vi "RX IQ Processing.vi"(0 "configuration":T4={"primary channel selector"=0.0, "last OFDM symbol index"=0, "switch format detection states"=TRUE, "format"=enum."NON_HT_OFDM", "bandwidth"=enum."20MHz"}, 1 "packet start":bool, 5 "channels in":T2, 9 "input valid":bool) -> (3 "primary channel selector":fxp<+,2,0>, 4 "last OFDM symbol index":u16, 6 "subcarrier index unsigned":u8, 8 "channel estimate timing":T3, 10 "channel estimate":T1, 12 "last sample":bool, 13 "subcarrier index":fxp<+/-,9,9>, 15 "output valid":bool=TRUE)   [LabVIEW 2020]
uses:
  Configuration Control.ctl
panel:
  out "subcarrier channel 2.Imag":fxp<+/-,25,4>
  out "subcarrier channel.Real":fxp<+/-,25,4>
  out "OFDM symbol start 2":bool
  out "packet_start 2":bool
  out "valid 2":bool
  out "OFDM symbol index 2":u16
  out "sample index 2":u16
  out "Imag 4":fxp<+/-,16,3>
  out "Real 4":fxp<+/-,16,3>
  out "OFDM symbol start":bool
  out "packet_start":bool
  out "valid":bool
  out "OFDM symbol index":u16
  out "sample index":u16
  out "Imag 3":fxp<+/-,16,3>
  out "Real 3":fxp<+/-,16,3>
  out "Imag 2":fxp<+/-,16,3>
  out "Real 2":fxp<+/-,16,3>
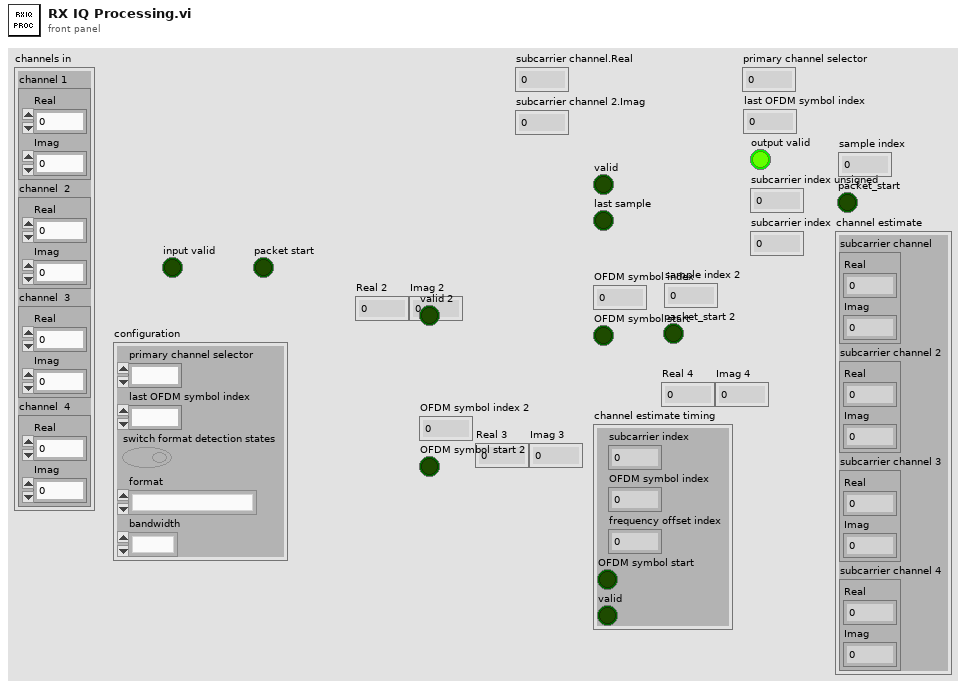
[diagram p1: front panel]
types:
  T1 = cluster{"subcarrier channel":cluster{"Real":fxp<+/-,25,4>, "Imag":fxp<+/-,25,4>}, "subcarrier channel 2":cluster{"Real":fxp<+/-,25,4>, "Imag":fxp<+/-,25,4>}, "subcarrier channel 3":cluster{"Real":fxp<+/-,25,4>, "Imag":fxp<+/-,25,4>}, "subcarrier channel 4":cluster{"Real":fxp<+/-,25,4>, "Imag":fxp<+/-,25,4>}}
  T2 = cluster{"channel 1 ":cluster{"Real":fxp<+/-,16,3>, "Imag":fxp<+/-,16,3>}, "channel  2":cluster{"Real":fxp<+/-,16,3>, "Imag":fxp<+/-,16,3>}, "channel  3":cluster{"Real":fxp<+/-,16,3>, "Imag":fxp<+/-,16,3>}, "channel  4":cluster{"Real":fxp<+/-,16,3>, "Imag":fxp<+/-,16,3>}}
  T3 = cluster{"subcarrier index":u8, "OFDM symbol index":u16, "frequency offset index":fxp<+/-,9,9>, "OFDM symbol start":bool, "valid":bool}
  T4 = typedef "Configuration Control.ctl" = cluster{"primary channel selector":fxp<+,2,0>, "last OFDM symbol index":u16, "switch format detection states":bool, "format":enum16{"NON_HT_OFDM", "VHT", "NON_HT_DUP_OFDM"}, "bandwidth":enum16{"20MHz", "40MHz", "80MHz"}}
  T5 = cluster{"sample index":u16, "OFDM symbol index":u16, "valid":bool, "packet_start":bool, "OFDM symbol start":bool}
  T6 = cluster{"L-STF-1":bool, "L-STF-2":bool, "L-LTF-1":bool, "L-LTF-2":bool, "L-SIG":bool, "L-Data":bool, "VHT-LTF":bool, "VHT-SIG-B":bool, "VHT-STF":bool, "VHT-Pilot":bool, "VHT-SIG-A-2":bool, "VHT-SIG-A-1":bool, "L-Pilot":bool, "VHT-Data":bool}
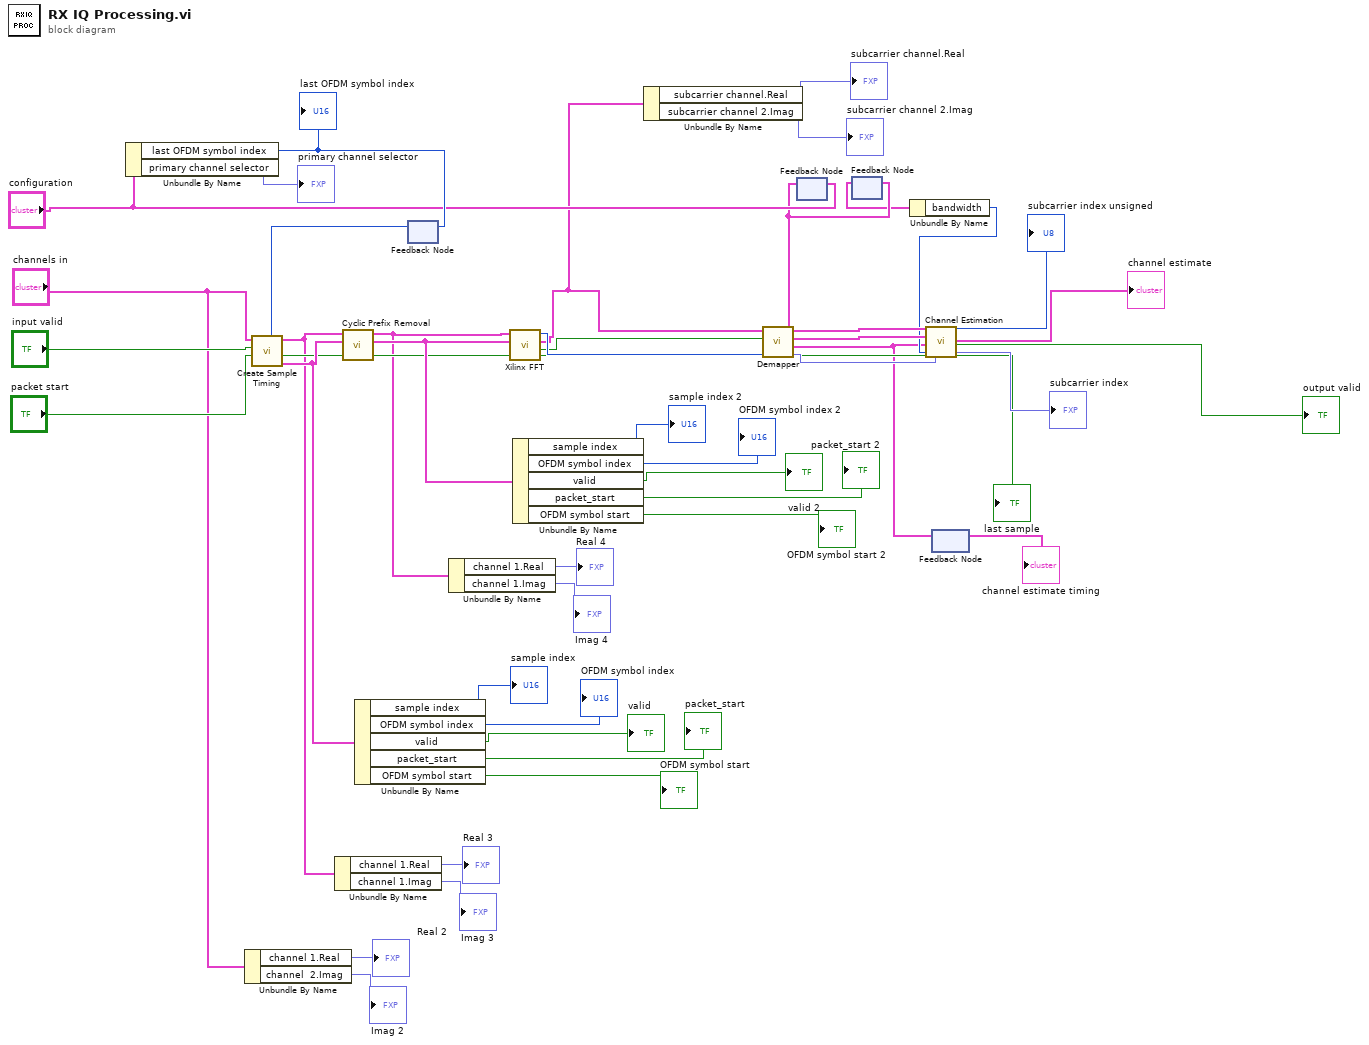
[diagram p0: block diagram]
diagram:
  n1 = Unbundle By Name("configuration") -> ("last OFDM symbol index"=w45:u16, "primary channel selector"=→"primary channel selector":fxp<+,2,0>)
  "last OFDM symbol index" <- w45
  n2 = Unbundle By Name("channels in") -> ("channel 1.Real"=→"Real 2":fxp<+/-,16,3>, "channel  2.Imag"=→"Imag 2":fxp<+/-,16,3>)
  n3 = feedback-in #1(w45) -> ()
  n4 = feedback #1() -> (w42:u16)  [unwired: 1 in]
  n5 = call "Create Sample Timing.vi"("Last OFDM symbol index"=w42, "packet start"="packet start", "input valid"="input valid", "channels in"="channels in") -> ("Cluster"=w26:T5, "last sample"=→"last sample":bool, "channels out"=w4:T2)  [unwired: 5 in]
  n6 = Unbundle By Name(w4) -> ("channel 1.Real"=→"Real 3":fxp<+/-,16,3>, "channel 1.Imag"=→"Imag 3":fxp<+/-,16,3>)
  n7 = call "Cyclic Prefix Removal.vi"("sample timing in"=w26, "channels in"=w4) -> ("sample timing out"=w13:T5, "channels out"=w3:T2)  [unwired: 8 in]
  n8 = Unbundle By Name(w26) -> ("sample index"=→"sample index":u16, "OFDM symbol index"=→"OFDM symbol index":u16, "valid"=→"valid":bool, "packet_start"=→"packet_start":bool, "OFDM symbol start"=→"OFDM symbol start":bool)
  n9 = Unbundle By Name(w3) -> ("channel 1.Real"=→"Real 4":fxp<+/-,16,3>, "channel 1.Imag"=→"Imag 4":fxp<+/-,16,3>)
  n10 = call "Xilinx FFT.vi"("sample timing"=w13, "channels in"=w3) -> ("output valid"=w38:bool, "subcarrier channels"=w2:T1, "OFDM symbol index"=w39:u16)  [unwired: 7 in]
  n11 = Unbundle By Name(w13) -> ("sample index"=→"sample index 2":u16, "OFDM symbol index"=→"OFDM symbol index 2":u16, "valid"=→"valid 2":bool, "packet_start"=→"packet_start 2":bool, "OFDM symbol start"=→"OFDM symbol start 2":bool)
  n12 = Unbundle By Name(w2) -> ("subcarrier channel.Real"=→"subcarrier channel.Real":fxp<+/-,25,4>, "subcarrier channel 2.Imag"=→"subcarrier channel 2.Imag":fxp<+/-,25,4>)
  n13 = feedback #2() -> (w37:T4)  [unwired: 1 in]
  n14 = call "Demapper.vi"("OFDM symbol index"=w39, "configuration"=w37, "input valid"=w38, "subcarrier channels"=w2) -> ("subcarrier index"=w10:fxp<+/-,9,9>, "subcarrier timing"=w7:T3, "field map"=w34:T6, "subcarrier channels out"=w35:T1)  [unwired: 4 in]
  n15 = feedback-in #2("configuration") -> ()
  n16 = feedback #3() -> (w36:T4)  [unwired: 1 in]
  n17 = feedback-in #3(w37) -> ()
  n18 = Unbundle By Name(w36) -> ("bandwidth"=w31:enum16{"20MHz", "40MHz", "80MHz"})
  n19 = call "Channel Estimation.vi"("subcarrier channels"=w35, "field map"=w34, "subcarrier timing"=w7, "bandwidth"=w31, "subcarrier index in"=w10) -> (20:"subcarrier index"=→"subcarrier index unsigned":u8, "channel estimate"=→"channel estimate":T1, "output valid"=→"output valid":bool, 26:"subcarrier index"=→"subcarrier index":fxp<+/-,9,9>)  [unwired: 19 in]
  n20 = feedback-in #4(w7) -> ()
  n21 = feedback #4() -> (→"channel estimate timing":T3)  [unwired: 1 in]
